vi "Serialize - JSON.vi"(8 "error in":errorcluster, 11 "MC Data in":refnum<class "MC Data.lvclass">) -> (0 "error out":errorcluster, 2 "Serialized JSON":string, 3 "MC Data out":refnum<class "MC Data.lvclass">)   [LabVIEW 2015, in "Alicat Lib.lvlib" / "MC Data.lvclass"]
uses:
  MC Data.lvclass
  MC Data.lvclass/MC Data.ctl
  Alicat Data.lvclass
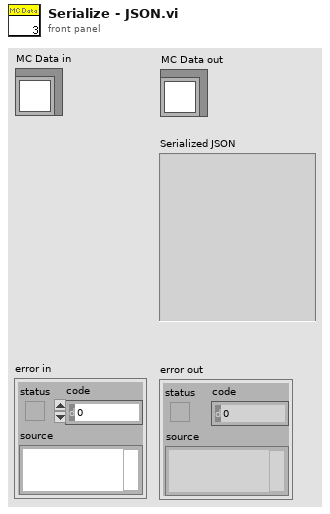
[diagram p1: front panel]
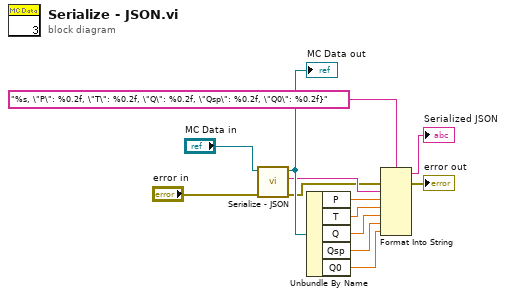
[diagram p0: block diagram]
diagram:
  n1 = call-parent "Serialize - JSON.vi"("error in"="error in", "Alicat Data in"="MC Data in") -> ("error out"=w2:errorcluster, "Serialized JSON"=w11:string, "Alicat Data out"=w13:refnum<class "MC Data.lvclass">)  [unwired: 7 in]
  "MC Data out" <- w13
  n2 = Unbundle By Name(w13) -> ("P"=w10:sgl, "T"=w9:sgl, "Q"=w8:sgl, "Qsp"=w7:sgl, "Q0"=w6:sgl)
  n3 = Format Into String(format string="%s, \"P\": %0.2f, \"T\": %0.2f, \"Q\": %0.2f, \"Qsp\": %0.2f, \"Q0\": %0.2f}", error in=w2, w11, w10, w9, w8, w7, w6) -> (resulting string=→"Serialized JSON":string, error out=→"error out":errorcluster)  [unwired: 1 in]
